vi "Gateway_Send.vi"(8 "error in (no error)":errorcluster, 10 "Send Data Via SSH Tunnel":bool, 11 "GatewayClass in":refnum<class "GatewayClass.lvclass">) -> (0 "error out":errorcluster, 2 "MIDAS Reply":string, 3 "GatewayClass out":refnum<class "GatewayClass.lvclass">)   [LabVIEW 2018, in "GatewayClass.lvclass"]
uses:
  GatewayClass.lvclass
  GatewayClass.lvclass/GatewayClass.ctl
  DataPacker/Utilities/SSH_TUNNEL.lvclass
panel:
  out "bytes written":i32
  out "GEM Bank Size":i32
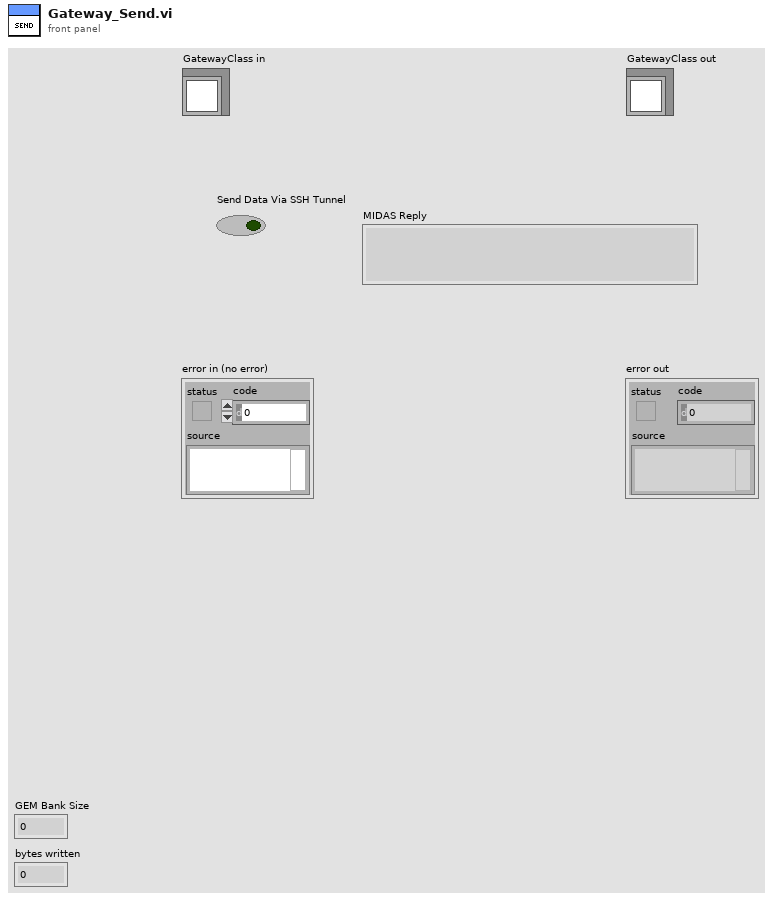
[diagram p1: front panel]
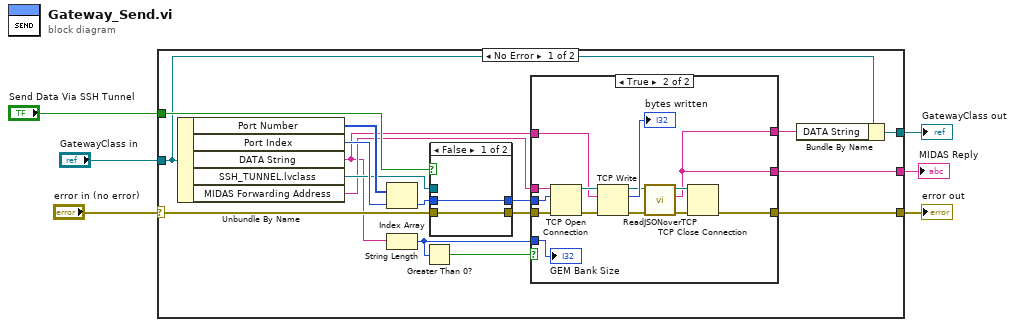
[diagram p0: block diagram]
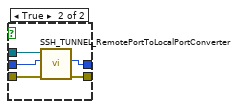
[diagram p2: hidden frame]
diagram:
  n1 = case shown="No Error" "error in (no error)" {
    selector: "error in (no error)" -> [w17 w47]
    tunnel: [w11 w47] -> w5
    tunnel: [w13 w46] -> w3
    tunnel: "GatewayClass in" -> [w14 w46]
    tunnel: "Send Data Via SSH Tunnel" -> [w16 _]
    tunnel: [w7 _] -> w1
    frame No Error {
      n2 = Unbundle By Name(w14) -> ("Port Number"=w19:u16[], "Port Index"=w18:i32, "DATA String"=w8:string, "SSH_TUNNEL.lvclass"=w10:refnum<class "SSH_TUNNEL.lvclass">, "MIDAS Forwarding Address"=w9:string)
      n3 = Index Array(array=w19, index=w18) -> (element=w22:u16)
      n4 = String Length(string=w8) -> (length=w15:i32)
      n5 = Greater Than 0?(x=w15) -> (x > 0?=w20:bool)
      n6 = case shown="False" w16 {
        tunnel: w17 -> [w25 w28]
        tunnel: [w25 w27] -> w21
        tunnel: w22 -> [w24 w30]
        tunnel: [w24 w29] -> w23
        tunnel: w10 -> [_ w26]
        frame False {
        }
        frame True {
          n7 = call "SSH_TUNNEL_RemotePortToLocalPortConverter.vi"("error in (no error)"=w28, "Remote Port Number"=w30, "SSH_TUNNEL in"=w26) -> ("error out"=w27:errorcluster, "Local Port Number"=w29:u16)  [unwired: 6 in, 1 out]
        }
      }
      n8 = case shown="True" w20 {
        tunnel: w23 -> [_ w45]
        tunnel: w15 -> [_ w36]
        tunnel: [w31 w41] -> w11
        tunnel: [_ w32] -> w12
        tunnel: w21 -> [w31 w35]
        tunnel: w9 -> [_ w34]
        tunnel: w8 -> [_ w33]
        tunnel: [_ w32] -> w7
        frame False {
        }
        frame True {
          n9 = TCP Open Connection(address=w34, remote port or service name=w45, error in (no error)=w35) -> (connection ID=w42:refnum<k5>, error out=w43:errorcluster)  [unwired: 2 in]
          n10 = TCP Write(connection ID=w42, data in=w33, error in (no error)=w43) -> (connection ID out=w40:refnum<k5>, bytes written=→"bytes written":i32, error out=w39:errorcluster)  [unwired: 1 in]
          n11 = call "ReadJSONoverTCP.vi"("error out"=w39, "connection ID"=w40) -> ("error out"=w38:errorcluster, "JSON"=w32:string, "connection ID"=w37:refnum<k5>)  [unwired: 7 in]
          n12 = TCP Close Connection(connection ID=w37, error in (no error)=w38) -> (error out=w41:errorcluster)  [unwired: 1 in, 1 out]
          "GEM Bank Size" <- w36
        }
      }
      n13 = Bundle By Name(cluster=w14, "DATA String"=w12) -> (w13:refnum<class "GatewayClass.lvclass">)
    }
    frame Error {
    }
  }
  "error out" <- w5
  "GatewayClass out" <- w3
  "MIDAS Reply" <- w1
